vi "ChannelList_GetIDs.vi"(8 "error in (no error)":errorcluster, 11 "OXY_SCPI Reseource In":refnum<visa-resource-name>) -> (0 "error out":errorcluster, 1 "communication_data":T1, 2 "Channel ID List":string[](array[string]), 3 "OXY_SCPI Reseource Out":refnum<visa-resource-name>)   [LabVIEW 2018, in "OXYGEN.lvlib"]
doc: "Queries the ids of all channels."
uses:
  OXYGEN.lvlib
  TypeDefs/Cluster_RawCommData.ctl
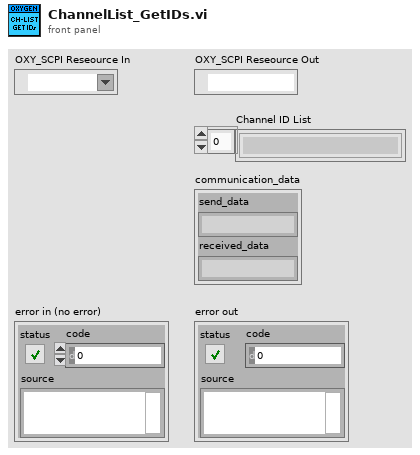
[diagram p1: front panel]
types:
  T1 = typedef "OXYGEN.lvlib/Cluster_RawCommData.ctl" = cluster{"send_data":string, "received_data":string}
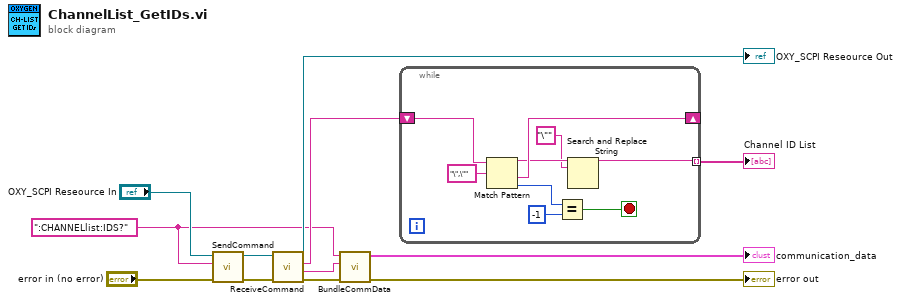
[diagram p0: block diagram]
diagram:
  w2 = ":CHANNELlist:IDS?"
  n1 = call "SendCommand.vi"("error in (no error)"="error in (no error)", "String to Send"=w2, "OXY_SCPI Reseource In"="OXY_SCPI Reseource In") -> ("error out"=w11:errorcluster, "OXY_SCPI Reseource Out"=w10:refnum<visa-resource-name>)  [unwired: 7 in]
  n2 = call "ReceiveCommand.vi"("error in (no error)"=w11, "OXY_SCPI Reseource In"=w10) -> ("error out"=w6:errorcluster, "received Data with Header"=w4:string, "received Data"=w3:string, "OXY_SCPI Reseource Out"=→"OXY_SCPI Reseource Out":refnum<visa-resource-name>)  [unwired: 6 in]
  n3 = call "BundleCommData.vi"("error in (no error)"=w6, "received_data"=w4, "send_data"=w2) -> ("error out"=→"error out":errorcluster, "communication_data"=→"communication_data":T1)  [unwired: 7 in]
  n4 = while {
    shift-right: [w16] -> _
    shift-left: w3 -> [w18]
    tunnel: [w13] -> w12 mode=indexing
    stop <- w19 stop-if-true
    n5 = Match Pattern(string=w18, regular expression="\",\"") -> (before substring=w15:string, after substring=w16:string, offset past match=w21:i32)  [unwired: 1 in, 1 out]
    n6 = Equal?(x=w21, y=-1) -> (x = y?=w19:bool)
    n7 = Search and Replace String(input string=w15, search string="\"" ("substring (\"\")")) -> (result string=w13:string)  [unwired: 6 in, 3 out]
  }
  "Channel ID List" <- w12
